vi "D32.vi"(2 "D":u32 format="%x", 3 "R":u32 format="%x", 4 "C":u32 format="%x") -> (0 "~Q":u32=4294967295 format="%x", 1 "Q":u32 format="%x")   [LabVIEW 2019, in "Triggers.lvlib"]
uses:
  Triggers.lvlib
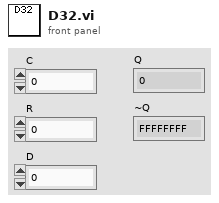
[diagram p1: front panel]
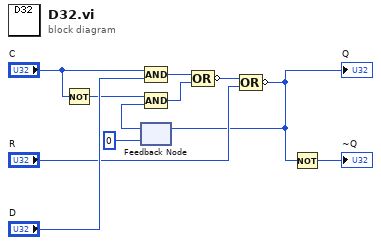
[diagram p0: block diagram]
diagram:
  n1 = Not(x="C") -> (.not. x?=w8:u32)
  n2 = feedback #1(u32 0) -> (w7:u32)
  n3 = Compound Arithmetic op=AND("C", "D") -> (w5:u32)
  n4 = Compound Arithmetic op=AND(w8, w7) -> (w4:u32)
  n5 = Compound Arithmetic op=OR(w5, w4) -> (invert w3:u32)
  n6 = Compound Arithmetic op=OR(w3, "R") -> (invert w1:u32)
  "Q" <- w1
  n7 = feedback-in #1(w1) -> ()
  n8 = Not(x=w1) -> (.not. x?=→"~Q":u32)
